vi "Servo setting.vi"   [LabVIEW 2016, in "Test2.lvrbt"]
uses:
  Test2.lvrbt
  <vilib>/NXT/Hardware/Plugins/Tetrix 180 deg Servo/Tetrix180ServoAddress.ctl
  <vilib>/NXT/NXTIO Xnodes/NXTIONodeSubVIs/TETRIX IO Move Servos.vi
  <vilib>/NXT/Dual Mode Library/Waits/Wait_Num.vi
  <vilib>/NXT/Subs/LVHSConnector.ctl
  <vilib>/NXT/NXTIO Xnodes/AddressXNode/NXTIOAddress.xnode
  <vilib>/NXT/NXTIO Xnodes/NXTIOXNode/NXTIO.xnode
  <vilib>/NXT/LegoClasses/BrickReference/BrickReference.lvclass
types:
  T1 = typedef "Tetrix180ServoAddress.ctl" = i32
  T2 = cluster{"Tetrix180Servo":T1, "Tetrix180Servo":T1, "Tetrix180Servo":T1, "Tetrix180Servo":T1, "Tetrix180Servo":T1, "Tetrix180Servo":T1}
  T3 = typedef "LVHSConnector.ctl" = refnum<class "BrickReference.lvclass">
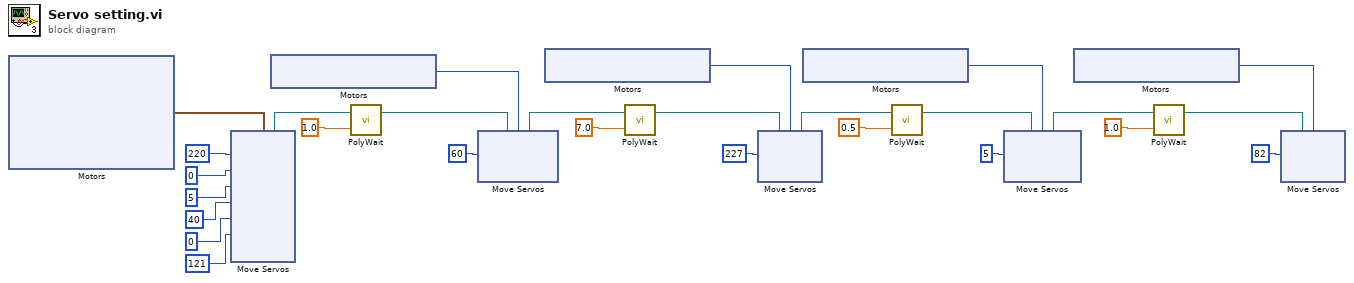
[diagram p0: block diagram]
diagram:
  n1 = xnode "Motors"() -> ("Motor"=w27:T2)
  n2 = xnode "Move Servos"("Position 6"=u8 121, "Position 5"=u8 0, "Position 4"=u8 40, "Position 3"=u8 5, "Position 2"=u8 0, "Position 1"=u8 220, "Motors"=w27) -> ("NXT/EV3"=w20:T3)  [unwired: 1 in]
  n3 = xnode "Motors"() -> ("Motor"=w19:T1)
  n4 = call-poly <vilib>:"PolyWait.vi"("Time (1 sec)"=sgl 1.0, "NXT/EV3"=w20) -> ("NXT/EV3"=w2:T3)  [unwired: 2 in]
  n5 = xnode "Move Servos"("Position 1"=u8 60, "Motors"=w19, "NXT/EV3"=w2) -> ("NXT/EV3"=w16:T3)
  n6 = xnode "Motors"() -> ("Motor"=w15:T1)
  n7 = call-poly <vilib>:"PolyWait.vi"("Time (1 sec)"=sgl 7.0, "NXT/EV3"=w16) -> ("NXT/EV3"=w13:T3)  [unwired: 2 in]
  n8 = xnode "Move Servos"("Position 1"=u8 227, "Motors"=w15, "NXT/EV3"=w13) -> ("NXT/EV3"=w11:T3)
  n9 = xnode "Motors"() -> ("Motor"=w10:T1)
  n10 = call-poly <vilib>:"PolyWait.vi"("Time (1 sec)"=sgl 0.5, "NXT/EV3"=w11) -> ("NXT/EV3"=w8:T3)  [unwired: 2 in]
  n11 = xnode "Move Servos"("Position 1"=u8 5, "Motors"=w10, "NXT/EV3"=w8) -> ("NXT/EV3"=w6:T3)
  n12 = xnode "Motors"() -> ("Motor"=w4:T1)
  n13 = call-poly <vilib>:"PolyWait.vi"("Time (1 sec)"=sgl 1.0, "NXT/EV3"=w6) -> ("NXT/EV3"=w3:T3)  [unwired: 2 in]
  n14 = xnode "Move Servos"("Position 1"=u8 82, "Motors"=w4, "NXT/EV3"=w3) -> ()  [unwired: 1 out]
